vi "Pockels Cal-Init.vi"(8 "error in (no error)":errorcluster, 11 "Pre-AOL Z wizard refs":T2) -> (0 "error out":errorcluster, 2 "Cal settings window's title":string, 3 "Initial state":T1)   [LabVIEW 2017]
uses:
  AOL Z/Typedefs/Pre-AOL Z wizard refs.ctl
  AOL Z/Typedefs/Cal mode.ctl
  Typedefs/Pockels cal wizard states.ctl
  Globals/gl_Calibration globals.vi
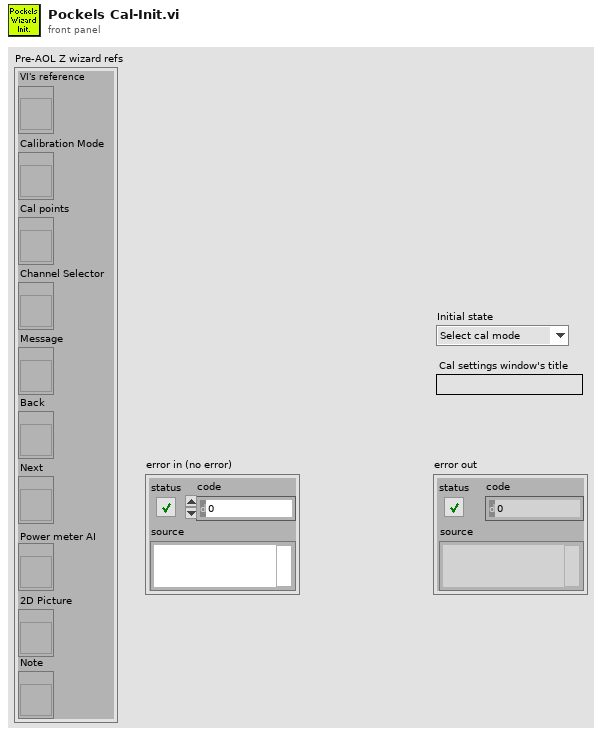
[diagram p1: front panel]
types:
  T1 = typedef "Pockels cal wizard states.ctl" = enum16{"Select cal mode", "Show instructions 1", "Select channel", "Show instructions 2", "Show instructions 3", "Confirm start", "Start calibration"}
  T2 = typedef "Pre-AOL Z wizard refs.ctl" = cluster{"VI's reference":refnum<vi>, "Calibration Mode":refnum<vi>, "Cal points":refnum<vi>, "Channel Selector":refnum<vi>, "Message":refnum<vi>, "Back":refnum<vi>, "Next":refnum<vi>, "Power meter AI":refnum<vi>, "2D Picture":refnum<vi>, "Note":refnum<vi>}
  T3 = typedef "Cal mode.ctl" = enum16{"Automatic", "Interactive"}
  T4 = enum8{"Enabled", "Disabled", "Disabled and Grayed Out"}
  T5 = typedef "LVRectTypeDef.ctl" = cluster{"Left":i16, "Top":i16, "Right":i16, "Bottom":i16}
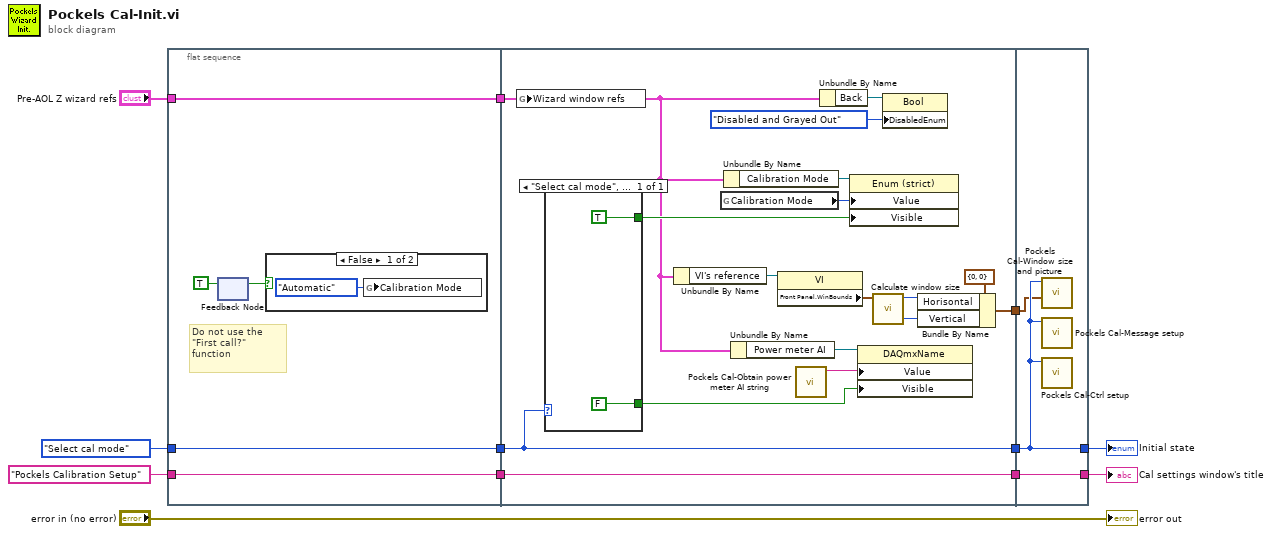
[diagram p0: block diagram]
diagram:
  n1 = flat-sequence {
    tunnel: "Pockels Calibration Setup" -> [w15]
    tunnel: Pockels_cal_wizard_states."Select cal mode" ("Initial state") -> [w16]
    tunnel: "Pre-AOL Z wizard refs" -> [w17]
    tunnel: [w17] -> w6
    tunnel: [w16] -> w5
    tunnel: [w15] -> w4
    tunnel: w6 -> [w24]
    tunnel: w5 -> [w28]
    tunnel: w4 -> [w27]
    tunnel: [w28] -> w3
    tunnel: [w27] -> w2
    tunnel: [w19] -> w1
    tunnel: [w40] -> w7
    tunnel: [w39] -> w9
    tunnel: w3 -> [w39]
    tunnel: w2 -> [w40]
    tunnel: w1 -> [w38]
    frame #0 {
      # "Do not use the \"First call?\" function"
      n2 = feedback #1() -> (w14:bool)  [unwired: 1 in]
      n3 = feedback-in #1(TRUE) -> ()
      n4 = case shown="False" w14 {
        frame False {
          n5 = global write "gl_Calibration globals.vi" "Calibration Mode"(Cal_mode."Automatic" ("Calibration Mode")) -> ()
        }
        frame True {
        }
      }
    }
    frame #1 {
      n6 = global write "gl_Calibration globals.vi" "Wizard window refs"(w24) -> ()
      n7 = case shown="\"Select cal mode\", Default" w28 {
        tunnel: [FALSE ("Visible")] -> w35
        tunnel: [TRUE ("Visible")] -> w34
        frame "Select cal mode", Default {
        }
      }
      n8 = Unbundle By Name(w24) -> ("VI's reference"=w25:refnum<vi>)
      n9 = global read "gl_Calibration globals.vi" "Calibration Mode"() -> (w33:T3)
      n10 = Unbundle By Name(w24) -> ("Calibration Mode"=w31:refnum<vi>)
      n11 = Unbundle By Name(w24) -> ("Power meter AI"=w32:refnum<vi>)
      n12 = property class="VI"(reference=w25) -> ("Front Panel.WinBounds"=w23:T5)  [unwired: 1 in, 2 out]
      n13 = call "Pockels Cal-Obtain power meter AI string.vi"() -> ("Power meter AI (string)"=w26:string)  [unwired: 10 in, 1 out]
      n14 = Unbundle By Name(w24) -> ("Back"=w30:refnum<vi>)
      n15 = property on="Property Node" class="Enum (strict)"(reference=w31, "Value"=w33, "Visible"=w34) -> ()  [unwired: 1 in, 2 out]
      n16 = property on="Property Node" class="DAQmxName"(reference=w32, "Value"=w26, "Visible"=w35) -> ()  [unwired: 1 in, 2 out]
      n17 = call "Calculate window size.vi"("Window bounds"=w23) -> ("Vertical window size"=w20:i16, "Horisontal window size"=w21:i16)  [unwired: 9 in]
      n18 = property on="Property Node" class="Bool"(reference=w30, "DisabledEnum"=T4."Disabled and Grayed Out" ("Disabled")) -> ()  [unwired: 1 in, 2 out]
      n19 = Bundle By Name(cluster=cluster{"Horisontal":i16, "Vertical":i16} {"Horisontal"=0, "Vertical"=0} ("Window size"), "Horisontal"=w21, "Vertical"=w20) -> (w19:cluster{"Horisontal":i16, "Vertical":i16})
    }
    frame #2 {
      n20 = call "Pockels Cal-Window size and picture.vi"("Original window size"=w38, "State"=w39) -> ()  [unwired: 9 in, 1 out]
      n21 = call "Pockels Cal-Message setup.vi"("State"=w39) -> ()  [unwired: 10 in, 1 out]
      n22 = call "Pockels Cal-Ctrl setup.vi"("State"=w39) -> ()  [unwired: 10 in, 1 out]
    }
  }
  "error out" <- "error in (no error)"
  "Initial state" <- w9
  "Cal settings window's title" <- w7
